vi "Main.vi"() -> ()   [LabVIEW 2021]
uses:
  Sub VIs/Trajectory Control/Trajectory_Control.ctl
  Sub VIs/Logging/Controller Data.ctl
  Sub VIs/Drive Motor/Drive Motor Data.ctl
  Sub VIs/Steering Motor/Steering Motor Data.ctl
  Sub VIs/State Estimator/State Estimate.ctl
  Sub VIs/State Estimator/Measurements.ctl
  Sub VIs/IMU/IMU Data.ctl
  Sub VIs/Steering Motor Encoder/Steering Motor Encoder Data.ctl
  Sub VIs/GNSS/GNSS Data.ctl
  <vilib>/Utility/RT CPU Load.ctl
  Sub VIs/Logging/Log Level.ctl
  <vilib>/Platform/TimedLoop/XDataNode/timing_clust.ctl
  <vilib>/Platform/TimedLoop/XDataNode/nitl_modes.ctl
  <vilib>/Platform/TimedLoop/XDataNode/wakeup.ctl
  Sub VIs/Steering Motor/Steering Motor Handle.ctl
  <vilib>/platform/TimedLoop/XDataNode/XDataNode.xnode
  <vilib>/Platform/TimedLoop/XDataNode/XDNodeRunTimeDep.lvlib
  <vilib>/NI_Real-Time Target Support.lvlib
panel:
  in  "Abort Trajectory":bool
  in  "Kp":dbl
  in  "Ki":dbl
  out "Speed":bool
  in  "?":bool
  out "RPM":bool
  in  "Drive Motor Speed (m/s)":dbl
  in  "file path (trajectorymat)":path=path "c:/ni-rt/startup/trajectorymat_asta0_line.csv"
  in  "file path (matrixmat)":path=path "c:/ni-rt/startup/matrixmat_default.csv"
  out "velocity":dbl(graph)
  out "CPU loads":T1[](array[typedef]) {"ISR (%)" format="%#.2f"; "Idle (%)" format="%#.2f"; "Background (%)" format="%#.2f"; "Normal (%)" format="%#.2f"; "Above Normal (%)" format="%#.2f"; "High (%)" format="%#.2g"; "Timed Structures (%)" format="%#.2g"; "Time Critical (%)" format="%#.2g"; "Total (%)" format="%#.2g"}
  out "Measurements (Debug)":T2 {"GNSS Data"."Longitude (deg)" format="%#.10g"; "GNSS Data"."Latitude (deg)" format="%#.10g"; "GNSS Data"."Longitude (rad)" format="%#_10g"; "GNSS Data"."Latitude (rad)" format="%#_10g"}
  out "State Estimate (Debug)":T6 {"Y (m)" format="%#_10g"; "X (m)" format="%#_10g"}
  out "Motor Controllers (Debug)":T7
  out "Trajectory (Debug)":T10
  out "State estimator Ts check":bool
  out "E2 limit hit":bool
  out "E1 limit hit":bool
  out "XY trajectory (0 is bikeposition)":T11(graph)
  out "Y-Offset":dbl
  out "X-Offset":dbl
  in  "Reset and Init trajectory":bool
  in  "Drive Motor Angular Speed (rad/s)":dbl
  in  "Enable Steering Motor":bool
  out "Steering Motor Enabled":bool
  out "Abort":bool
  in  "Reset Steering Motor Encoder":bool
  in  "Stop Button":bool
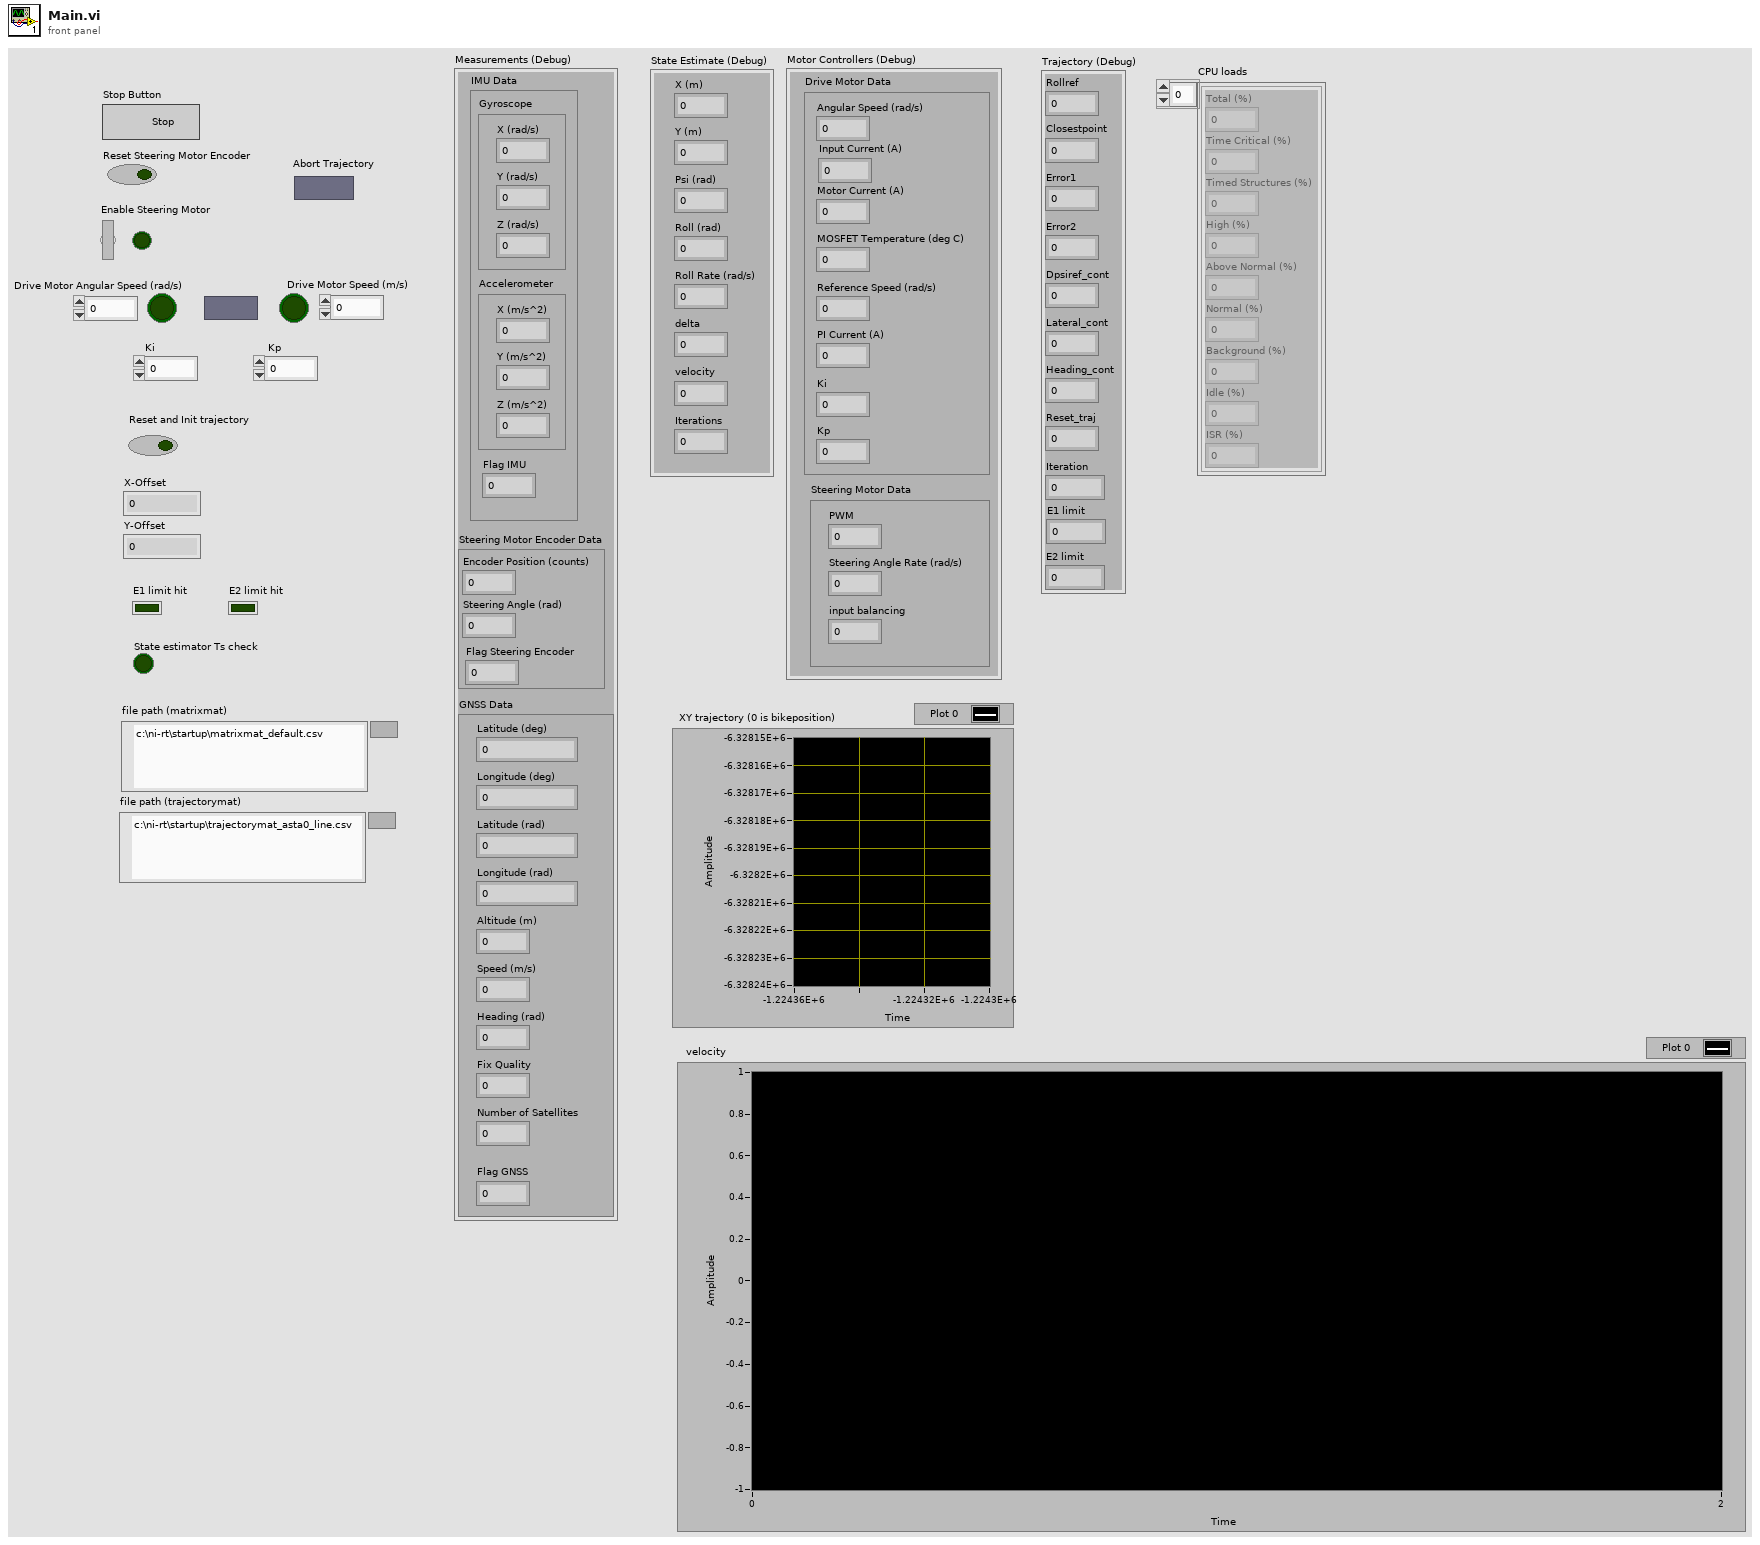
[diagram p1: front panel]
types:
  T1 = typedef "NI_Real-Time Target Support.lvlib/RT CPU Load.ctl" = cluster{"Total (%)":dbl, "Time Critical (%)":dbl, "Timed Structures (%)":dbl, "High (%)":dbl, "Above Normal (%)":dbl, "Normal (%)":dbl, "Background (%)":dbl, "Idle (%)":dbl, "ISR (%)":dbl}
  T2 = typedef "Measurements.ctl" = cluster{"IMU Data":T3, "Steering Motor Encoder Data":T4, "GNSS Data":T5}
  T3 = typedef "IMU Data.ctl" = cluster{"Gyroscope":cluster{"X (rad/s)":dbl, "Y (rad/s)":dbl, "Z (rad/s)":dbl}, "Accelerometer":cluster{"X (m/s^2)":dbl, "Y (m/s^2)":dbl, "Z (m/s^2)":dbl}, "Flag IMU":dbl}
  T4 = typedef "Steering Motor Encoder Data.ctl" = cluster{"Encoder Position (counts)":i32, "Steering Angle (rad)":dbl, "Flag Steering Encoder":dbl}
  T5 = typedef "GNSS Data.ctl" = cluster{"Latitude (rad)":dbl, "Longitude (rad)":dbl, "Altitude (m)":dbl, "Speed (m/s)":dbl, "Heading (rad)":dbl, "Fix Quality":i32, "Number of Satellites":i32, "Latitude (deg)":dbl, "Longitude (deg)":dbl, "Flag GNSS":dbl}
  T6 = typedef "State Estimate.ctl" = cluster{"X (m)":dbl, "Y (m)":dbl, "Psi (rad)":dbl, "Roll (rad)":dbl, "Roll Rate (rad/s)":dbl, "delta":dbl, "velocity":dbl, "Iterations":dbl}
  T7 = typedef "Controller Data.ctl" = cluster{"Drive Motor Data":T8, "Steering Motor Data":T9}
  T8 = typedef "Drive Motor Data.ctl" = cluster{"Angular Speed (rad/s)":dbl, "Input Current (A)":dbl, "Motor Current (A)":dbl, "MOSFET Temperature (deg C)":dbl, "Reference Speed (rad/s)":dbl, "PI Current (A)":dbl, "Ki":dbl, "Kp":dbl}
  T9 = typedef "Steering Motor Data.ctl" = cluster{"PWM":dbl, "Steering Angle Rate (rad/s)":dbl, "input balancing":dbl}
  T10 = typedef "Trajectory_Control.ctl" = cluster{"Rollref":dbl, "Closestpoint":dbl, "Error1":dbl, "Error2":dbl, "Dpsiref_cont":dbl, "Lateral_cont":dbl, "Heading_cont":dbl, "Reset_traj":dbl, "Iteration":dbl, "E1 limit":u32, "E2 limit":u32}
  T11 = cluster{"Trajectory(X/Y/PSI)":dbl[], "Trajectory(X/Y/PSI)":dbl[]}
  T12 = cluster{"Steering Angle Rate":dbl, "rollReference":dbl, "roll":dbl, "rollRate":dbl, "Kp":dbl, "Kd":dbl, "steering_flag":i32}
  T13 = typedef "XDNodeRunTimeDep.lvlib/timing_clust.ctl" = cluster{"Expected End [f-1]":u64, "Actual End [f-1]":u64, "Finished Late? [f-1]":bool, "Expected End [i-1]":u64, "Actual End [i-1]":u64, "Finished Late? [i-1]":bool, "Expected Start [i]":u64, "Actual Start [i]":u64, "Expected Start [f]":u64, "Actual Start [f]":u64, "Source Name":string, "Structure Name":string, "Period":i64, "Deadline":i64, "Offset":i64, "Start":i64, "Priority":i32, "Timeout":i32, "Mode":T14, "Wakeup Reason":T15, "Error":errorcluster, "Source Type":string, "Secondary Source Type":string, "Global End Time":u64, "Global Start Time":u64, "Frame Duration":u64, "Iteration Duration":u64, "Assigned CPU":i32, "I/O Scan Engine Mode":u32}
  T14 = typedef "XDNodeRunTimeDep.lvlib/nitl_modes.ctl" = enum32{"No Change", "Process missed periods, maintain original phase", "Discard missed periods, maintain original phase", "Process missed periods, ignore original phase", "Discard missed periods, ignore original phase"}
  T15 = typedef "XDNodeRunTimeDep.lvlib/wakeup.ctl" = enum32{"Normal", "Aborted", "Asynchronous wakeup", "Timing source error", "Timed loop error", "Timeout"}
  T16 = typedef "Steering Motor Handle.ctl" = cluster{"Dummy":dbl}
  T17 = typedef "Log Level.ctl" = enum16{"Error", "Warning", "Info"}
  T18 = cluster{"B":dbl[], "A":dbl[][], "C":dbl[][], "D":dbl[], "K":dbl[][], "Trajectory":dbl[][], "Init":dbl[], "parameter":dbl[][]}
  T19 = typedef "Configuration.ctl" = cluster{"Accelerometer Bias":cluster{"X (m/s)":dbl, "Y (m/s)":dbl, "Z (m/s)":dbl}, "Gyroscope Bias":cluster{"X (m/s)":dbl, "Y (m/s)":dbl, "Z (m/s)":dbl}, "Steering Motor Gear Ratio":dbl, "Steering Pully Gear Ratio":dbl, "Steering Encoder CPR":dbl, "Steering Motor Max RPM":dbl, "Wheelbase (m)":dbl, "Fork Angle (rad)":dbl, "Balancing Controller":cluster{"Kp (/s)":dbl, "Kd (1)":dbl}, "Max Allowed Steering Angle (rad)":dbl, "Task Periods":cluster{"Emergency Stop (us)":i64, "IMU (us)":i64, "Steering Motor Encoder (us)":i64, "State Estimator (us)":i64, "Balancing Controller (us)":i64, "GNSS (us)":i64, "Logging (us)":i64, "Drive Motor (us)":i64, "Visualization (us)":i64}, "Drive Motor Gear Ratio":dbl, "lr":dbl, "lf":dbl, "lambda":dbl, "k1":dbl, "k2":dbl, "e1_max":dbl, "Ad_t":dbl, "Bd_t":dbl, "C_t":dbl, "D_t":dbl, "Wheel radius":dbl}
  T20 = typedef "NI_Matrix.lvlib/RealMatrix.ctl" = dbl[][]
  T21 = typedef "IMU Handle.ctl" = cluster{"I2C address":u8}
  T22 = typedef "GNSS Handle.ctl" = cluster{"VISA Resource Name":refnum<visa-resource-name>}
  T23 = typedef "Drive Motor Handle.ctl" = cluster{"VISA Resource Name":refnum<visa-resource-name>}
  T24 = typedef "Log Handle.ctl" = cluster{"Data File":refnum<file>, "Event File":refnum<file>}
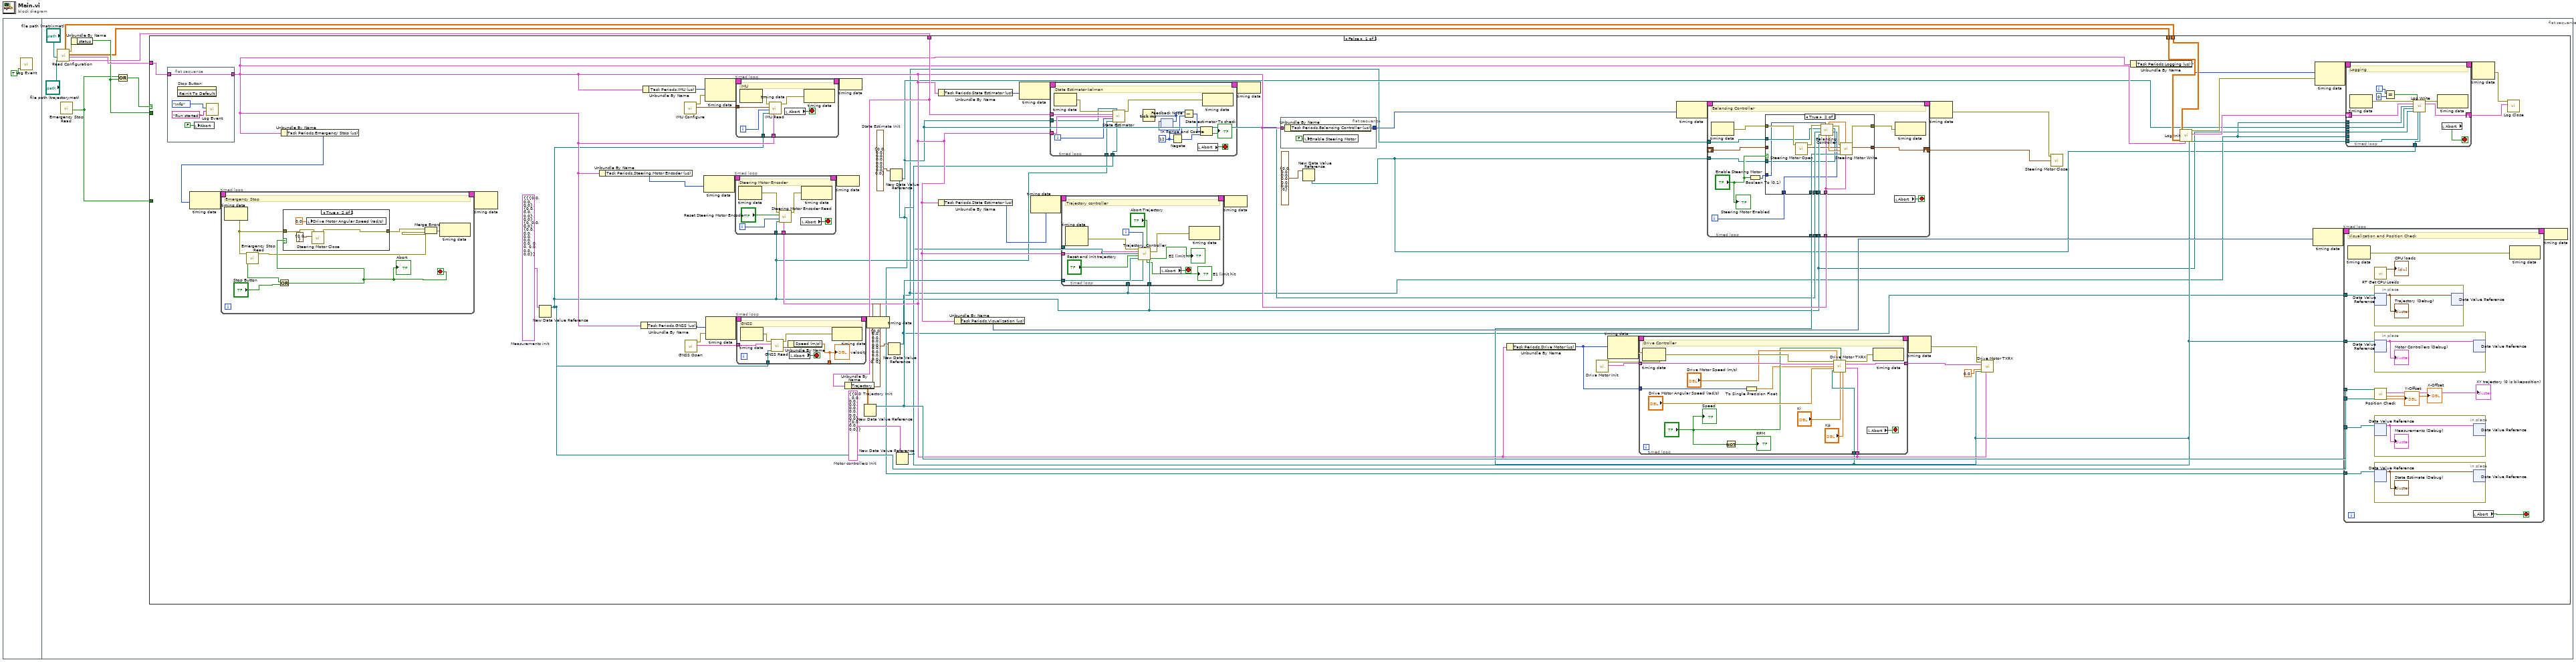
[diagram p0: block diagram]
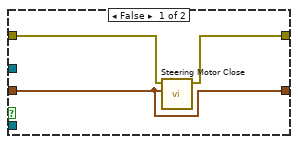
[diagram p2: hidden frame]
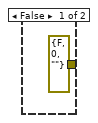
[diagram p3: hidden frame]
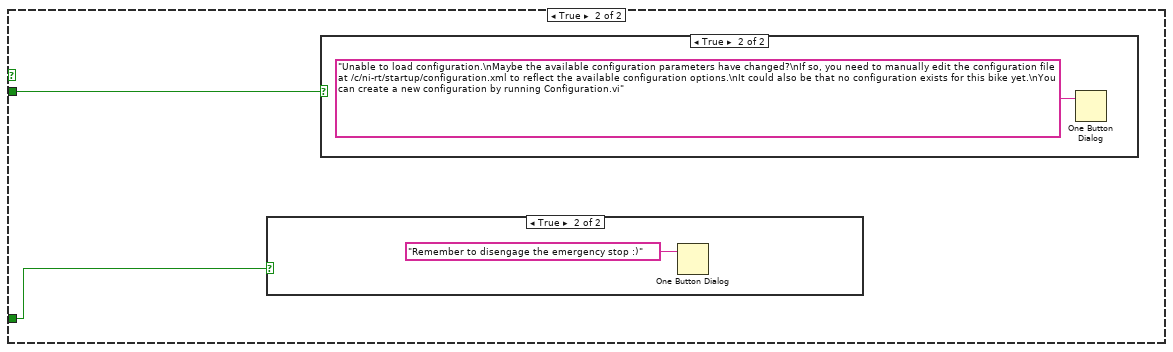
[diagram p4: hidden frame]
diagram:
  n1 = flat-sequence {
    frame #0 {
      n2 = call "Log Event.vi"("Clear Log"=TRUE) -> ()  [unwired: 10 in, 1 out]
    }
    frame #1 {
      n3 = call "Read Configuration.vi"("file path (trajectorymat)"="file path (trajectorymat)", "file path (matrixmat)"="file path (matrixmat)") -> ("values loded in xml files"=w9:T18, "configuration"=w11:T19, "value"=w4:T20, "error out"=w10:errorcluster, "Init trajectory (2)"=w6:dbl[][])  [unwired: 3 in, 2 out]
      n4 = call "Emergency Stop Read.vi"() -> ("Emergency Stop"=w7:bool)  [unwired: 10 in, 1 out]
      n5 = Unbundle By Name(w10) -> ("status"=w8:bool)
      n6 = Compound Arithmetic op=OR(w7, w8) -> (w5:bool)
      n7 = case shown="False" w5 {
        tunnel: w8 -> [_ w317]
        tunnel: w11 -> [w51 _]
        tunnel: w9 -> [w24 _]
        tunnel: w7 -> [_ w316]
        tunnel: w6 -> [w43 _]
        tunnel: w4 -> [w26 _]
        frame False {
          w32 = T10 {"Rollref"=0.0, "Closestpoint"=0.0, "Error1"=0.0, "Error2"=0.0, "Dpsiref_cont"=0.0, "Lateral_cont"=0.0, "Heading_cont"=0.0, "Reset_traj"=0.0, "Iteration"=0.0, "E1 limit"=0, "E2 limit"=0}  # Trajectory Init
          w44 = T6 {"X (m)"=0.0, "Y (m)"=0.0, "Psi (rad)"=0.0, "Roll (rad)"=0.0, "Roll Rate (rad/s)"=0.0, "delta"=0.0, "velocity"=0.0, "Iterations"=0.0}  # State Estimate Init
          w50 = T7 {"Drive Motor Data"={"Angular Speed (rad/s)"=0.0, "Input Current (A)"=0.0, "Motor Current (A)"=0.0, "MOSFET Temperature (deg C)"=0.0, "Reference Speed (rad/s)"=0.0, "PI Current (A)"=0.0, "Ki"=0.0, "Kp"=0.0}, "Steering Motor Data"={"PWM"=0.0, "Steering Angle Rate (rad/s)"=0.0, "input balancing"=0.0}}  # Motor controllers Init
          w73 = T2 {"IMU Data"={"Gyroscope"={"X (rad/s)"=0.0, "Y (rad/s)"=0.0, "Z (rad/s)"=0.0}, "Accelerometer"={"X (m/s^2)"=0.0, "Y (m/s^2)"=0.0, "Z (m/s^2)"=0.0}, "Flag IMU"=0.0}, "Steering Motor Encoder Data"={"Encoder Position (counts)"=0, "Steering Angle (rad)"=0.0, "Flag Steering Encoder"=0.0}, "GNSS Data"={"Latitude (rad)"=0.0, "Longitude (rad)"=0.0, "Altitude (m)"=0.0, "Speed (m/s)"=0.0, "Heading (rad)"=0.0, "Fix Quality"=0, "Number of Satellites"=0, "Latitude (deg)"=0.0, "Longitude (deg)"=0.0, "Flag GNSS"=0.0}}  # Measurements init
          n8 = flat-sequence {
            tunnel: [w312] -> w23
            tunnel: w51 -> [w312]
            frame #0 {
              n9 = invoke on="Stop Button" class="Bool (strict)" method="Reinit To Default"() -> ()  [unwired: 3 in, 3 out]
              n10 = local write "Abort"(FALSE ("Abort")) -> ()
              n11 = call "Log Event.vi"("Message"="Run started!", "Log Level"=Log_Level."Info") -> ()  [unwired: 9 in, 1 out]
            }
          }
          n12 = Unbundle By Name(w23) -> ("Task Periods.Emergency Stop (us)"=w72:i64)
          n13 = node-c288(w72) -> (w71:T13)
          n14 = timed-loop {
            timing: w71 -> [_]
            timing-out: [_] -> w70
            stop <- w295 stop-if-true
            # "Emergency Stop"
            n15 = node-c288() -> (w297:errorcluster)  [unwired: 1 in]
            n16 = call "Emergency Stop Read.vi"("Error In"=w297) -> ("Emergency Stop"=w292:bool, "Error Out"=w293:errorcluster)  [unwired: 9 in]
            n17 = Or(x=w292, y="Stop Button") -> (x .or. y?=w295:bool)
            "Abort" <- w295
            n18 = case shown="True" w295 {
              tunnel: w297 -> [_ w302]
              tunnel: [errorcluster {"status"=FALSE, "code"=0, "source"=""} ("Error Out") w301] -> w294
              frame False {
              }
              frame True {
                n19 = local write "Drive Motor Angular Speed (rad/s)"(0.0 ("Drive Motor Angular Speed (rad/s)")) -> ()
                n20 = call "Steering Motor Close.vi"("Steering Motor Handle"=T16 {"Dummy"=0.0}, "Error In"=w302) -> ("Error Out"=w301:errorcluster)  [unwired: 9 in]
              }
            }
            n21 = Merge Errors(w294, w293) -> (w296:errorcluster)
            n22 = node-c288(w296) -> ()  [unwired: 1 out]
          }
          n23 = node-c288(w70) -> ()  [unwired: 1 out]
          n24 = New Data Value Reference(data value=w73) -> (data value reference=w19:refnum<data-value>)  [unwired: 1 in, 1 out]
          n25 = Unbundle By Name(w23) -> ("Task Periods.Steering Motor Encoder (us)"=w56:i64)
          n26 = Unbundle By Name(w23) -> ("Task Periods.GNSS (us)"=w53:i64)
          n27 = Unbundle By Name(w23) -> ("Task Periods.IMU (us)"=w57:i64)
          n28 = call "IMU Configure.vi"() -> ("IMU Handle"=w58:T21, "Error Out"=w59:errorcluster)  [unwired: 10 in]
          n29 = call "GNSS Open.vi"() -> ("GNSS Handle"=w54:T22, "Error Out"=w55:errorcluster)  [unwired: 10 in]
          n30 = node-c288(w56) -> (w63:T13)
          n31 = node-c288(w57, w59) -> (w65:T13)
          n32 = node-c288(w53, w55) -> (w61:T13)
          n33 = timed-loop {
            timing: w63 -> [_]
            timing-out: [_] -> w62
            tunnel: w19 -> [w214]
            tunnel: w23 -> [w212]
            i -> [w213]
            stop <- w215 stop-if-true
            # "Steering Motor Encoder"
            n34 = node-c288() -> (w218:errorcluster)  [unwired: 1 in]
            n35 = call "Steering Motor Encoder Read.vi"("Configuration"=w212, "Measurement In"=w214, "Flag Steering Encoder"=w213, "Reset Counter"="Reset Steering Motor Encoder", "Error In"=w218) -> ("Error Out"=w217:errorcluster)  [unwired: 4 in, 2 out]
            n36 = local read "Abort"() -> (w215:bool)
            n37 = node-c288(w217) -> ()  [unwired: 1 out]
          }
          n38 = timed-loop {
            timing: w65 -> [_]
            timing-out: [_] -> w64
            tunnel: w58 -> [w232]
            tunnel: w19 -> [w230]
            tunnel: w23 -> [w229]
            i -> [w228]
            stop <- w231 stop-if-true
            # "IMU"
            n39 = node-c288() -> (w234:errorcluster)  [unwired: 1 in]
            n40 = call "IMU Read.vi"("Configuration"=w229, "Measurement In"=w230, "Flag IMU"=w228, "IMU Handle"=w232, "Error In"=w234) -> ("Error Out"=w233:errorcluster)  [unwired: 4 in, 2 out]
            n41 = local read "Abort"() -> (w231:bool)
            n42 = node-c288(w233) -> ()  [unwired: 1 out]
          }
          n43 = timed-loop {
            timing: w61 -> [_]
            timing-out: [_] -> w60
            tunnel: w54 -> [w201]
            tunnel: w19 -> [w197]
            tunnel: [w195] -> _
            stop <- w198 stop-if-true
            # "GNSS"
            n44 = node-c288() -> (w200:errorcluster)  [unwired: 1 in]
            n45 = call "GNSS Read.vi"("Measurement In"=w197, "GNSS Handle"=w201, "Error In"=w200) -> ("GNSS Data"=w196:T5, "Error Out"=w199:errorcluster)  [unwired: 6 in, 1 out]
            n46 = Unbundle By Name(w196) -> ("Speed (m/s)"=w195:dbl)
            "velocity" <- w195
            n47 = local read "Abort"() -> (w198:bool)
            n48 = node-c288(w199) -> ()  [unwired: 1 out]
          }
          n49 = node-c288(w62) -> ()
          n50 = node-c288(w64) -> ()
          n51 = Unbundle By Name(w24) -> ("Trajectory"=w31:dbl[][])
          n52 = New Data Value Reference(data value=w31) -> (data value reference=w25:refnum<data-value>)  [unwired: 1 in, 1 out]
          n53 = node-c288(w60) -> ()
          n54 = New Data Value Reference(data value=w32) -> (data value reference=w17:refnum<data-value>)  [unwired: 1 in, 1 out]
          n55 = New Data Value Reference(data value=w44) -> (data value reference=w18:refnum<data-value>)  [unwired: 1 in, 1 out]
          n56 = New Data Value Reference(data value=w50) -> (data value reference=w20:refnum<data-value>)  [unwired: 1 in, 1 out]
          n57 = Unbundle By Name(w23) -> ("Task Periods.State Estimator (us)"=w21:i64)
          n58 = Unbundle By Name(w23) -> ("Task Periods.State Estimator (us)"=w33:i64)
          n59 = Unbundle By Name(w23) -> ("Task Periods.Visualization (us)"=w27:i64)
          n60 = node-c288(w21) -> (w35:T13)
          n61 = node-c288(w33) -> (w13:T13)
          n62 = timed-loop {
            timing: w35 -> [_]
            timing-out: [_] -> w34
            tunnel: w19 -> [w129]
            tunnel: w24 -> [w132]
            tunnel: w20 -> [w128]
            tunnel: w18 -> [w127]
            tunnel: w23 -> [w131]
            i -> [w130]
            stop <- w135 stop-if-true
            w121 = i64 12 ("y")
            # "State Estimator kalman"
            n63 = node-c288() -> (w134:errorcluster)  [unwired: 1 in]
            n64 = call "State Estimator.vi"("Error In"=w134, "State Estimate In"=w127, "Matrix"=w132, "Configuration"=w131, "Iteration"=w130, "Measurement In"=w129, "Balancing controller In"=w128) -> ("Error out"=w133:errorcluster)  [unwired: 7 in, 1 out]
            n65 = Tick Count (ms)() -> (millisecond timer value=w126:u32)
            n66 = feedback-in #1(w126) -> ()
            n67 = feedback #1() -> (w125:u32)  [unwired: 1 in]
            n68 = Negate(x=w121) -> (-x=w122:i64)
            n69 = Subtract(x=w126, y=w125) -> (x-y=w123:u32)
            n70 = local read "Abort"() -> (w135:bool)
            n71 = In Range and Coerce(upper limit=w121, x=w123, lower limit=w122) -> (In Range?=→"State estimator Ts check":bool)  [unwired: 1 out]
            n72 = node-c288(w133) -> ()  [unwired: 1 out]
          }
          n73 = timed-loop {
            timing: w13 -> [_]
            timing-out: [_] -> w12
            tunnel: w18 -> [w85]
            tunnel: w23 -> [w82]
            tunnel: w19 -> [w80]
            tunnel: w25 -> [w79]
            tunnel: w17 -> [w77]
            i -> [w81]
            stop <- w86 stop-if-true
            # "Trajectory controller"
            n74 = node-c288() -> (w83:errorcluster)  [unwired: 1 in, 1 out]
            n75 = call "Trajectory_Controller.vi"("Error In"=w83, "reset"=w81, "Abort Trajectory"="Abort Trajectory", "Configuration"=w82, "State Estimate In"=w85, "Reset and Init trajectory"="Reset and Init trajectory", "RefTraj in"=w79, "Trajectory In"=w77, "Measurement In"=w80) -> ("Error out"=w84:errorcluster, "E1 limit"=→"E1 limit hit":bool, "E2 limit"=→"E2 limit hit":bool)  [unwired: 2 in, 2 out]
            n76 = local read "Abort"() -> (w86:bool)
            n77 = node-c288(w84) -> ()  [unwired: 1 out]
          }
          n78 = node-c288(w12) -> ()
          n79 = node-c288(w34) -> ()
          n80 = flat-sequence {
            tunnel: [w246] -> w52
            tunnel: w23 -> [w245]
            frame #0 {
              n81 = Unbundle By Name(w245) -> ("Task Periods.Balancing Controller (us)"=w246:i64)
              n82 = local write "Enable Steering Motor"(FALSE ("Enable Steering Motor")) -> ()
            }
          }
          n83 = New Data Value Reference(data value=T12 {"Steering Angle Rate"=0.0, "rollReference"=0.0, "roll"=0.0, "rollRate"=0.0, "Kp"=0.0, "Kd"=0.0, "steering_flag"=0} ("output cluster")) -> (data value reference=w15:refnum<data-value>)  [unwired: 1 in, 1 out]
          n84 = Unbundle By Name(w23) -> ("Task Periods.Drive Motor (us)"=w14:i64)
          n85 = call "Drive Motor Init.vi"() -> ("Drive Motor Handle"=w40:T23, "Error Out"=w39:errorcluster)  [unwired: 10 in]
          n86 = node-c288(w14, w39) -> (w42:T13)
          n87 = timed-loop {
            timing: w42 -> [_]
            timing-out: [_] -> w41
            tunnel: w40 -> [w157]
            tunnel: w23 -> [w153]
            tunnel: w20 -> [w154]
            tunnel: [w158] -> w36
            tunnel: w14 -> [w145]
            stop <- w159 stop-if-true
            # "Drive Controller"
            n88 = node-c288() -> (w156:errorcluster)  [unwired: 1 in]
            n89 = Not(x="?") -> (.not. x?=→"RPM":bool)
            n90 = To Single Precision Float(number=w145) -> (single precision float=w146:sgl)
            n91 = call "Drive Motor TXRX.vi"("Error In"=w156, "Speed Control (m/s)"="Drive Motor Speed (m/s)", "RPM / Speed"="?", "Drive Motor Handle In"=w157, "Tasking Period"=w146, "RPM Control (rad/s)"="Drive Motor Angular Speed (rad/s)", "Controller Data In"=w154, 12:w153, "Ki"="Ki", "Kp"="Kp") -> ("Error Out"=w155:errorcluster, "Drive Motor Handle Out"=w158:T23)  [unwired: 2 in, 2 out]
            n92 = local read "Abort"() -> (w159:bool)
            n93 = node-c288(w155) -> ()  [unwired: 1 out]
            "Speed" <- "?"
          }
          n94 = node-c288(w52) -> (w69:T13)
          n95 = timed-loop {
            timing: w69 -> [_]
            timing-out: [_] -> w68
            tunnel: w18 -> [w257]
            tunnel: w19 -> [w256]
            shift-right: [w258] -> w67
            shift-left: _ -> [w255]
            tunnel: w23 -> [w254]
            tunnel: w20 -> [w253]
            tunnel: w17 -> [w252]
            tunnel: w15 -> [w249]
            i -> [w248]
            stop <- w261 stop-if-true
            # "Balancing Controller"
            n96 = node-c288() -> (w260:errorcluster)  [unwired: 1 in]
            n97 = Boolean To (0,1)(Boolean="Enable Steering Motor") -> (0, 1=w250:i16)
            n98 = case shown="True" "Enable Steering Motor" {
              tunnel: w260 -> [w264 w274]
              tunnel: [w263 w279] -> w259
              tunnel: [w262 w278] -> w258
              tunnel: w257 -> [_ w276]
              tunnel: w256 -> [_ w275]
              tunnel: w255 -> [w262 _]
              tunnel: w254 -> [_ w270]
              tunnel: w253 -> [_ w271]
              tunnel: w252 -> [_ w269]
              tunnel: w250 -> [_ w267]
              tunnel: w249 -> [_ w266]
              tunnel: w248 -> [_ w265]
              frame False {
                n99 = call "Steering Motor Close.vi"("Steering Motor Handle"=w262, "Error In"=w264) -> ("Error Out"=w263:errorcluster)  [unwired: 9 in]
              }
              frame True {
                n100 = call "Steering Motor Open.vi"("Error In"=w274) -> ("Steering Motor Handle"=w272:T16, "Error Out"=w273:errorcluster)  [unwired: 9 in]
                n101 = call "Balancing Controller.vi"("t"=w265, "Balance In"=w266, "Configuration"=w270, "steering indicator flag"=w267, "Measurement In"=w275, "State Estimate In"=w276, "Trajectory In"=w269, "Error In"=w273) -> ("Error Out"=w280:errorcluster, "Steering Angle Rate (rad/s)"=w277:dbl, "Input balancing"=w268:dbl)  [unwired: 1 out]
                n102 = call "Steering Motor Write.vi"("Configuration"=w270, "Input balancing"=w268, "Controller Data In"=w271, "Steering Angle Rate (rad/s)"=w277, "Steering Motor Handle In"=w272, "Error In"=w280) -> ("Steering Motor Handle Out"=w278:T16, "Error Out"=w279:errorcluster)  [unwired: 2 in, 2 out]
              }
            }
            n103 = local read "Abort"() -> (w261:bool)
            n104 = node-c288(w259) -> ()  [unwired: 1 out]
            "Steering Motor Enabled" <- "Enable Steering Motor"
          }
          n105 = node-c288(w41) -> (w38:errorcluster)
          n106 = node-c288(w68) -> (w66:errorcluster)
          n107 = call "Drive Motor TXRX.vi"("Error In"=w38, "Drive Motor Handle In"=w36, "RPM Control (rad/s)"=0.0 ("Angular Speed (rad/s)"), "Controller Data In"=w20, 12:w23) -> ()  [unwired: 7 in, 4 out]
          n108 = call "Steering Motor Close.vi"("Steering Motor Handle"=w67, "Error In"=w66) -> ()  [unwired: 9 in, 1 out]
          n109 = Unbundle By Name(w23) -> ("Task Periods.Logging (us)"=w22:i64)
          n110 = call "Log Init.vi"("Configuration"=w23, "Matrices"=w26, "Trajectory"=w43) -> ("Log Handle"=w45:T24, "Error Out"=w47:errorcluster)  [unwired: 7 in]
          n111 = node-c288(w27) -> (w29:T13)
          n112 = node-c288(w22, w47) -> (w49:T13)
          n113 = timed-loop {
            timing: w29 -> [_]
            timing-out: [_] -> w28
            tunnel: w25 -> [w106]
            tunnel: w19 -> [w105]
            tunnel: w20 -> [w101]
            tunnel: w19 -> [w100]
            tunnel: w18 -> [w99]
            tunnel: w17 -> [w98]
            stop <- w96 stop-if-true
            # "Visualization and Position Check"
            n114 = node-c288() -> (w107:errorcluster)  [unwired: 1 in]
            n115 = call <vilib>:"RT Get CPU Loads.vi"() -> ("CPU loads"=→"CPU loads":T1[])  [unwired: 10 in, 1 out]
            n116 = in-place {
              n117 = in-place-dvr #2(w98) -> (w108:T10)  [unwired: 1 out]
              "Trajectory (Debug)" <- w108
              n118 = in-place-dvr #2(w108) -> ()  [unwired: 2 out]
            }
            n119 = in-place {
              n120 = in-place-dvr #3(w101) -> (w109:T7)  [unwired: 1 out]
              "Motor Controllers (Debug)" <- w109
              n121 = in-place-dvr #3(w109) -> ()  [unwired: 2 out]
            }
            n122 = call "Position Check.vi"("data value reference 2"=w105, "data value reference"=w106) -> ("Y-Offset"=→"Y-Offset":dbl, "X-Offset"=→"X-Offset":dbl, "XY Graph"=→"XY trajectory (0 is bikeposition)":T11)  [unwired: 7 in]
            n123 = in-place {
              n124 = in-place-dvr #4(w100) -> (w111:T2)  [unwired: 1 out]
              "Measurements (Debug)" <- w111
              n125 = in-place-dvr #4(w111) -> ()  [unwired: 2 out]
            }
            n126 = in-place {
              n127 = in-place-dvr #5(w99) -> (w110:T6)  [unwired: 1 out]
              "State Estimate (Debug)" <- w110
              n128 = in-place-dvr #5(w110) -> ()  [unwired: 2 out]
            }
            n129 = local read "Abort"() -> (w96:bool)
            n130 = node-c288(w107) -> ()  [unwired: 1 out]
          }
          n131 = timed-loop {
            timing: w49 -> [_]
            timing-out: [_] -> w48
            tunnel: w19 -> [w173]
            tunnel: w18 -> [w176]
            shift-right: [w178] -> w30
            shift-left: w45 -> [w177]
            tunnel: w20 -> [w175]
            tunnel: w17 -> [w174]
            tunnel: w17 -> [_]
            tunnel: w15 -> [w171]
            i -> [w172]
            stop <- w183 stop-if-true
            # "Logging"
            n132 = node-c288() -> (w180:errorcluster)  [unwired: 1 in]
            n133 = Equal?(x=w172, y=0) -> (x = y?=w181:bool)
            n134 = call "Log Write.vi"("Error In"=w180, "Write Header"=w181, "Log Handle In"=w177, "Trajectory In"=w174, "State Estimate In"=w176, "Measurement In"=w173, "Controller Data In"=w175, "Balance In"=w171) -> ("Error Out"=w179:errorcluster, "Log Handle Out"=w178:T24)  [unwired: 1 in, 5 out]
            n135 = node-c288(w179) -> ()  [unwired: 1 out]
            n136 = local read "Abort"() -> (w183:bool)
          }
          n137 = node-c288(w48) -> (w46:errorcluster)
          n138 = call "Log Close.vi"("Log Handle In"=w30, "Error In"=w46) -> ()  [unwired: 9 in, 1 out]
          n139 = node-c288(w28) -> ()
        }
        frame True {
          n140 = case shown="True" w316 {
            frame False {
            }
            frame True {
              n141 = One Button Dialog(message="Remember to disengage the emergency stop :)") -> ()  [unwired: 1 in, 1 out]
            }
          }
          n142 = case shown="True" w317 {
            frame False {
            }
            frame True {
              n143 = One Button Dialog(message="Unable to load configuration.\nMaybe the available configuration parameters have changed?\nIf so, you need to manually edit the configuration file at /c/ni-rt/startup/configuration.xml to reflect the available configuration options.\nIt could also be that no configuration exists for this bike yet.\nYou can create a new configuration by running Configuration.vi") -> ()  [unwired: 1 in, 1 out]
            }
          }
        }
      }
    }
  }
